vi "Cascade (SubVI).vi"(11 "FreqFspec in":T1(array[cluster])) -> (3 "3D Plot lvclass Array out":refnum<class "3D Plot Datatype.lvclass">[](array[class]))   [LabVIEW 2012]
uses:
  <vilib>/Math Plots/3D Math Plots/3D Plot/3D Plot Datatype/3D Plot Datatype.lvclass
  <vilib>/Math Plots/3D Math Plots/3D Surface/3D Surface Datatype/Public/Plot Helper (Vector).vi
  <vilib>/Math Plots/3D Math Plots/3D Surface/3D Surface Datatype/3D Surface Datatype.lvclass
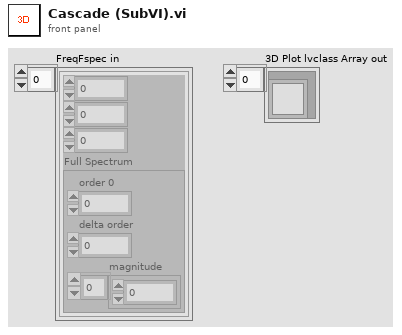
[diagram p1: front panel]
types:
  T1 = cluster{dbl, dbl, dbl, "Full Spectrum":cluster{"order 0":dbl, "delta order":dbl, "magnitude":dbl[]}}[]
  T2 = cluster{"order 0":dbl, "delta order":dbl, "magnitude":dbl[]}
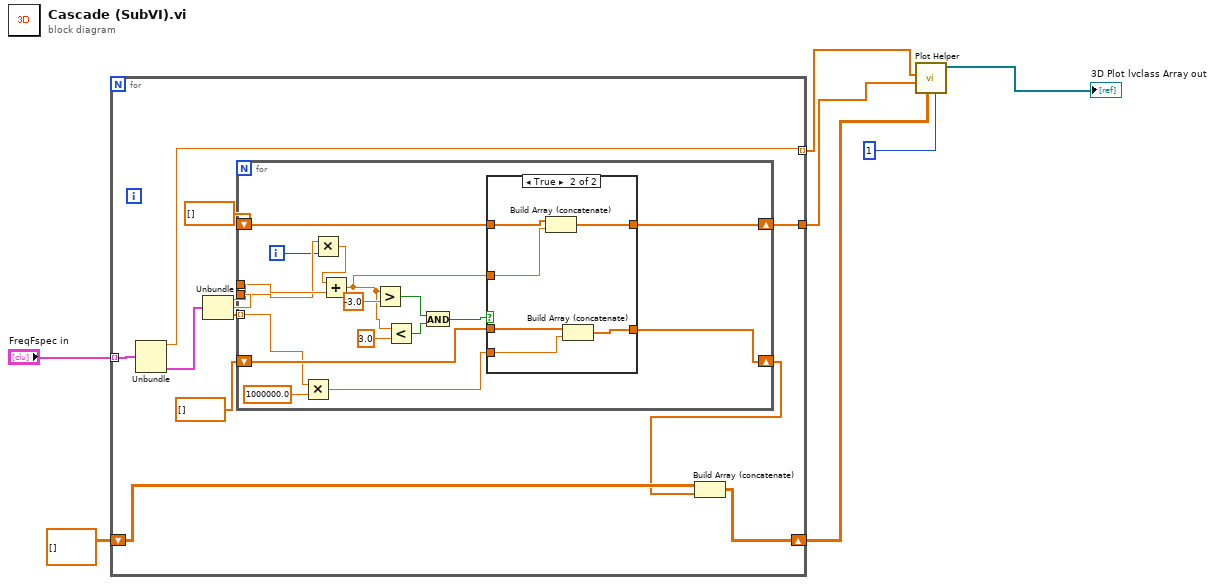
[diagram p0: block diagram]
diagram:
  n1 = for {
    shift-right: [w14] -> w4
    shift-left: sgl[][] [] ("z matrix") -> [w13]
    tunnel: "FreqFspec in" -> [w19] mode=indexing
    tunnel: [w11] -> w2 mode=indexing
    tunnel: [w10] -> w1
    n2 = Unbundle(w19) -> (w11:dbl, "Full Spectrum"=w18:T2)  [unwired: 2 out]
    n3 = Unbundle(w18) -> ("order 0"=w15:dbl, "delta order"=w16:dbl, "magnitude"=w17:dbl[])
    n4 = for {
      tunnel: w17 -> [w21] mode=indexing
      tunnel: w16 -> [w30]
      tunnel: w15 -> [w31]
      shift-right: [w25] -> w8
      shift-left: dbl[] [] ("magnitude") -> [w26]
      shift-right: [w24] -> w10
      shift-left: dbl[] [] ("magnitude") -> [w23]
      i -> [w29]
      n5 = Multiply(x=w21, y=1000000.0) -> (x*y=w22:dbl)
      n6 = Multiply(x=w30, y=w29) -> (x*y=w32:dbl)
      n7 = Add(x=w32, y=w31) -> (x+y=w27:dbl)
      n8 = Greater?(x=w27, y=-3.0) -> (0:w35:bool)
      n9 = Less?(x=w27, y=3.0) -> (x < y?=w36:bool)
      n10 = And(x=w35, y=w36) -> (x .and. y?=w28:bool)
      n11 = case shown="True" w28 {
        tunnel: w22 -> [_ w44]
        tunnel: w27 -> [_ w39]
        tunnel: w26 -> [w38 w43]
        tunnel: [w38 w42] -> w25
        tunnel: [w37 w41] -> w24
        tunnel: w23 -> [w37 w40]
        frame False {
        }
        frame True {
          n12 = Build Array (concatenate)(w40, w39) -> (w41:dbl[])
          n13 = Build Array (concatenate)(w43, w44) -> (w42:dbl[])
        }
      }
    }
    n14 = Build Array (concatenate)(w13, w8) -> (w14:dbl[][])
  }
  n15 = call-poly <vilib>:"Plot Helper.vi"("Plot ID"=1, "z matrix"=w4, "y vector"=w1, "x vector"=w2) -> ("3D Plot lvclass Array out"=→"3D Plot lvclass Array out":refnum<class "3D Plot Datatype.lvclass">[])  [unwired: 3 in, 4 out]
